vi "Take ADC Samples.vi"(8 "error in":errorcluster, 9 "Wait":i32, 10 "Iterations":i32, 11 "PAS In":T1 caption="Gas") -> (0 "error out":errorcluster, 2 "standard deviation":dbl, 3 "PAS Out":T1 caption="Gas", 5 "mean":dbl format="%0.2f")   [LabVIEW 2015]
uses:
  CAN Communication/PAS/Typedefs/Session Handle.ctl
  CAN Communication/PAS/PAS.lvclass
  <vilib>/Analysis/NI_AALBase.lvlib
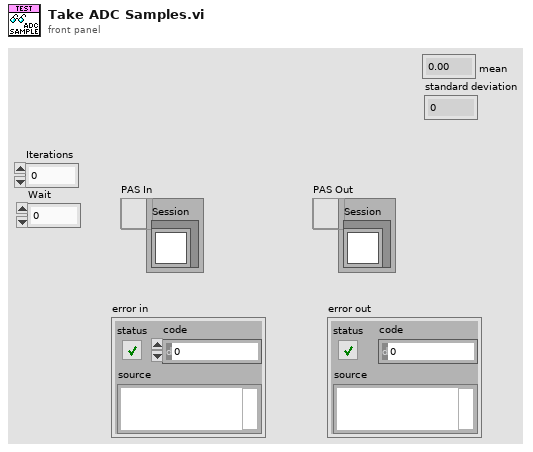
[diagram p1: front panel]
types:
  T1 = typedef "PAS.lvclass/Session Handle.ctl" = refnum<data-value>
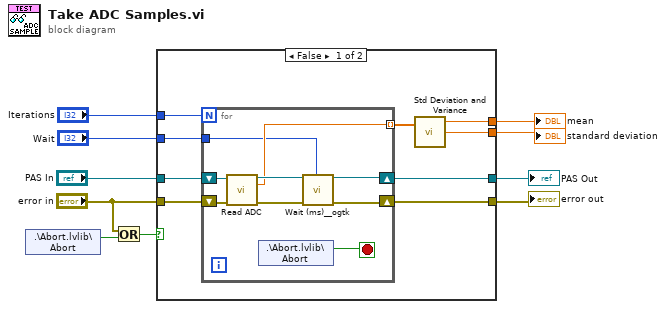
[diagram p0: block diagram]
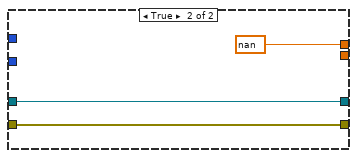
[diagram p2: hidden frame]
diagram:
  n1 = shared-variable ".\\Abort.lvlib\\Abort"() -> (w3:bool)  [unwired: 1 in, 1 out]
  n2 = Or(x="error in", y=w3) -> (x .or. y?=w4:bool)
  n3 = case shown="False" w4 {
    tunnel: [w19 nan ("mean")] -> w10
    tunnel: "PAS In" -> [w17 w29]
    tunnel: "error in" -> [w16 w28]
    tunnel: [w15 w29] -> w8
    tunnel: [w14 w28] -> w7
    tunnel: "Iterations" -> [w13 _]
    tunnel: "Wait" -> [w12 _]
    tunnel: [w11 _] -> w1
    frame False {
      n4 = for {
        N: w13 -> [_]
        shift-right: [w23] -> w14
        shift-left: w16 -> [w26]
        shift-right: [w25] -> w15
        shift-left: w17 -> [w27]
        tunnel: [w22] -> w18 mode=indexing
        tunnel: w12 -> [w21]
        stop <- w20 stop-if-true
        n5 = call "Read ADC.vi"("Session Handle in"=w27, "error in (no error)"=w26) -> ("Session Handle out"=w25:T1, "ADC"=w22:dbl, "error out"=w24:errorcluster)  [unwired: 9 in, 2 out]
        n6 = shared-variable ".\\Abort.lvlib\\Abort"() -> (w20:bool)  [unwired: 1 in, 1 out]
        n7 = call <userlib>:"Wait (ms)__ogtk.vi"("error in (no error)"=w24, "milliseconds to wait"=w21) -> ("error out"=w23:errorcluster)  [unwired: 8 in, 1 out]
      }
      n8 = call <vilib>:"Std Deviation and Variance.vi"("X"=w18) -> ("mean"=w19:dbl, "standard deviation"=w11:dbl)  [unwired: 1 in, 1 out]
    }
    frame True {
    }
  }
  "mean" <- w10
  "PAS Out" <- w8
  "error out" <- w7
  "standard deviation" <- w1
